vi "setID.vi"(8 "error in (no error)":errorcluster, 10 "ID":u32, 11 "GraphSearch in":refnum<class "GraphSearch.lvclass">) -> (0 "error out":errorcluster, 3 "GraphSearch out":refnum<class "GraphSearch.lvclass">)   [LabVIEW 2009, in "GraphSearch.lvclass"]
uses:
  GraphSearch.lvclass
  GraphSearch.lvclass/GraphSearch.ctl
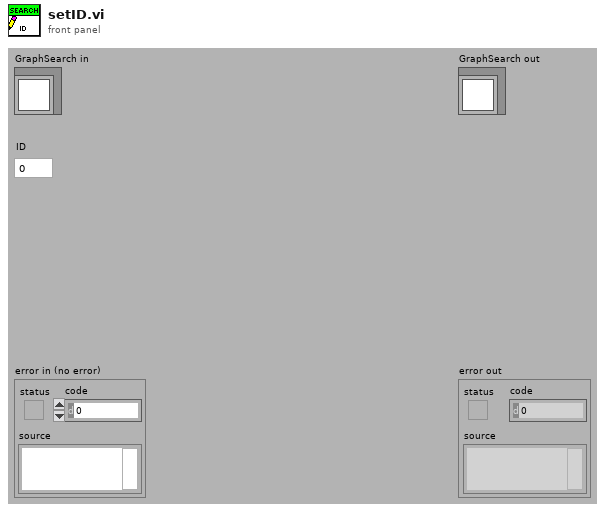
[diagram p1: front panel]
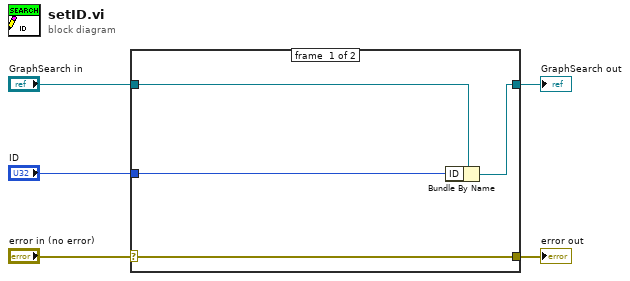
[diagram p0: block diagram]
diagram:
  n1 = case shown="No Error" "error in (no error)" {
    selector: "error in (no error)" -> [w9 w10]
    tunnel: [w9 w10] -> w4
    tunnel: [w7 w11] -> w2
    tunnel: "GraphSearch in" -> [w8 w11]
    tunnel: "ID" -> [w6 _]
    frame #0 {
      n2 = Bundle By Name(cluster=w8, "ID"=w6) -> (w7:refnum<class "GraphSearch.lvclass">)
    }
    frame #1 {
    }
  }
  "error out" <- w4
  "GraphSearch out" <- w2
